vi "stage distance mode.vi"(7 "LabVIEW error IN":errorcluster, 9 "Pos":dbl, 10 "XPS Reference IN":refnum<k24>) -> (0 "LabVIEW error OUT":errorcluster, 2 "Enable error":i32, 3 "XPS Reference OUT":refnum<k24>)   [LabVIEW 2015]
uses:
  D:/labview program/whole brain TP_221122_xz/sub vi/XPS-UNIFIED/LabVIEW VIs/LabVIEW Source Code/Dll/Newport.XPS.CommandInterface.dll
  XPS-UNIFIED/LabVIEW VIs/LabVIEW Source Code/Dll/Newport.XPS.CommandInterface.dll
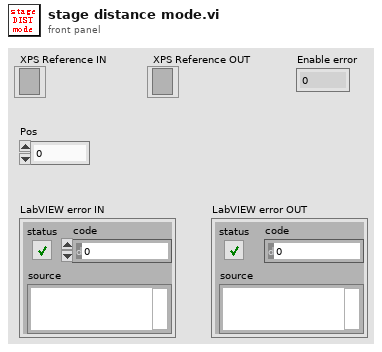
[diagram p1: front panel]
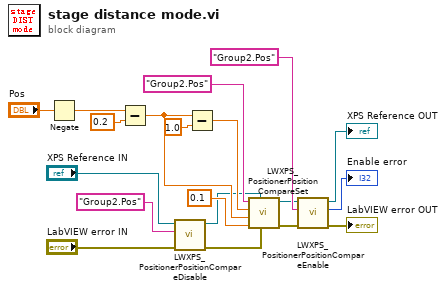
[diagram p0: block diagram]
diagram:
  n1 = Negate(x="Pos") -> (-x=w11:dbl)
  n2 = Subtract(x=w11, y=0.2) -> (x-y=w9:dbl)
  n3 = call "LWXPS_PositionerPositionCompareDisable.vi"("LabVIEW error IN"="LabVIEW error IN", "Positioner Name"="Group2.Pos", "CommandInterfaceXPS.XPS"="XPS Reference IN") -> ("LabVIEW error OUT"=w5:errorcluster, "CommandInterfaceXPS.XPS"=w3:refnum<k24>)  [unwired: 3 in, 2 out]
  n4 = Subtract(x=w9, y=1.0) -> (x-y=w10:dbl)
  n5 = call "LWXPS_PositionerPositionCompareSet.vi"("LabVIEW error IN"=w5, "CommandInterfaceXPS.XPS"=w3, "Position Step"=0.1, "Maximum Position"=w9, "Minimum Position"=w10, "Positioner Name"="Group2.Pos") -> ("LabVIEW error OUT"=w1:errorcluster, "CommandInterfaceXPS.XPS"=w2:refnum<k24>)  [unwired: 1 in, 2 out]
  n6 = call "LWXPS_PositionerPositionCompareEnable.vi"("LabVIEW error IN"=w1, "Positioner Name"="Group2.Pos", "CommandInterfaceXPS.XPS"=w2) -> ("LabVIEW error OUT"=→"LabVIEW error OUT":errorcluster, "Returned error code"=→"Enable error":i32, "CommandInterfaceXPS.XPS"=→"XPS Reference OUT":refnum<k24>)  [unwired: 3 in, 1 out]
